vi "ConfigureNetworkAdapterByMAC.vi"(8 "error in (no error)":errorcluster, 10 "Network Adapter Settings":T1={"Adapter Mode"=1, "IsPrimary"=FALSE, "MACAddr"="", "IP Address Request Mode"=1, "IPAddr"="", "SubnetMask"="", "Gateway"="", "DNSServer"="", "Alias"=""} {"IP Address Request Mode" items=["Static"=1, "DHCP/Link Local"=2, "Link-Local Only"=4, "DHCP Only"=8]; "Adapter Mode" items=["Disabled"=1, "TCP/IP Ethernet"=2, "Deterministic"=4, "EtherCAT"=8, "TCP/IP WLAN Connect"=32, "TCP/IP WLAN Create"=64]}, 11 "Session in":refnum<k21>="localhost") -> (0 "error out":errorcluster, 2 "requires restart":bool, 3 "Session out":refnum<k21>)   [LabVIEW 2017, in "SystemInfoProcess.lvlib"]
uses:
  <vilib>/addons/SystemInfoProcess/SystemInfoProcess.lvlib
  <vilib>/addons/SystemInfoProcess/controls/NetworkAdapterSettings.ctl
  <vilib>/nisyscfg/Find Hardware.vi
  <vilib>/nisyscfg/Save Changes (Hardware).vi
  <vilib>/nisyscfg/Close (Hardware).vi
  <vilib>/nisyscfg/Close (Filter).vi
  <vilib>/nisyscfg/nisyscfg.lvlib
  <resource>/objmgr/niflexriosae.rc
  <resource>/objmgr/nicriosae.rc
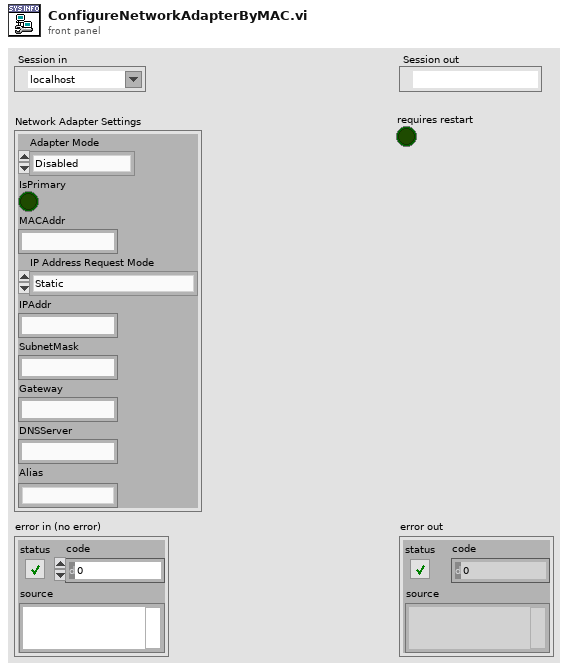
[diagram p1: front panel]
types:
  T1 = typedef "SystemInfoProcess.lvlib/NetworkAdapterSettings.ctl" = cluster{"Adapter Mode":u32, "IsPrimary":bool, "MACAddr":string, "IP Address Request Mode":u32, "IPAddr":string, "SubnetMask":string, "Gateway":string, "DNSServer":string, "Alias":string}
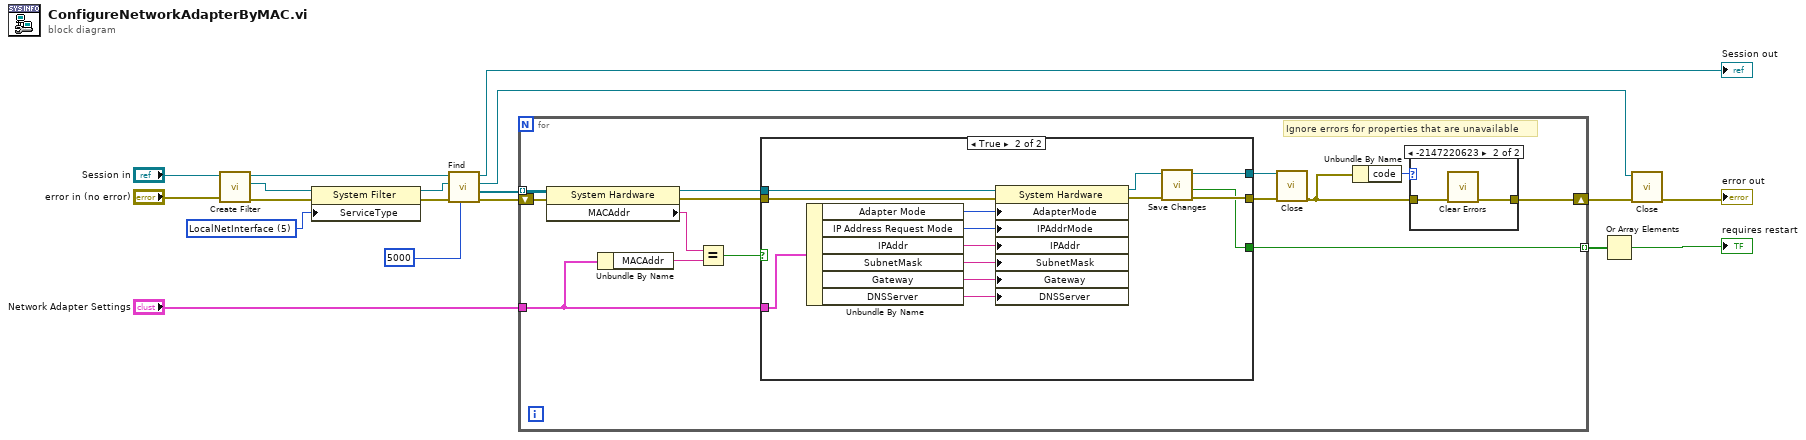
[diagram p0: block diagram]
diagram:
  w17 = u32 5 items=["mDnsNiTcp", "mDnsNiRealtime", "mDnsNiSysapi", "mDnsNiHttp", "LocalSystem", "LocalNetInterface", "LocalTimeKeeper", "LocalTimeSource", "mDnsLxi"] ("Service Type")
  n1 = call <vilib>:"Create Filter.vi"("error in (no error)"="error in (no error)", "Session in"="Session in") -> ("error out"=w16:errorcluster, "Filter out"=w18:refnum<k20>, "Session out"=w14:refnum<k21>)  [unwired: 7 in]
  n2 = property class="System Filter"(reference=w18, error in=w16, "ServiceType"=w17) -> (reference out=w13:refnum<k20>, error out=w15:errorcluster)
  n3 = call-poly <vilib>:"Find.vi"("Remote Timeout (300,000 ms)"=u32 5000 ("Timeout (milliseconds)"), "error in (no error)"=w15, "Filter in"=w13, "Session in"=w14) -> ("error out"=w11:errorcluster, "Resources out"=w12:refnum<k20>[], "Filter out"=w10:refnum<k20>, "Session out"=→"Session out":refnum<k21>)  [unwired: 4 in]
  n4 = for {
    tunnel: w12 -> [w31] mode=indexing
    shift-right: [w29] -> w8
    shift-left: w11 -> [w32]
    tunnel: "Network Adapter Settings" -> [w23]
    tunnel: [w19] -> w9 mode=indexing
    # "Ignore errors for properties that are unavailable"
    n5 = property class="System Hardware"(reference=w31, error in=w32) -> (reference out=w28:refnum<k20>, error out=w27:errorcluster, "MACAddr"=w26:string)
    n6 = Unbundle By Name(w23) -> ("MACAddr"=w25:string)
    n7 = Equal?(x=w26, y=w25) -> (x = y?=w24:bool)
    n8 = case shown="True" w24 {
      tunnel: w28 -> [w34 w48]
      tunnel: w27 -> [w33 w47]
      tunnel: [w34 w36] -> w21
      tunnel: [w33 w37] -> w22
      tunnel: w23 -> [_ w46]
      tunnel: [_ w35] -> w19
      frame False {
      }
      frame True {
        n9 = Unbundle By Name(w46) -> ("Adapter Mode"=w45:u32, "IP Address Request Mode"=w44:u32, "IPAddr"=w43:string, "SubnetMask"=w42:string, "Gateway"=w41:string, "DNSServer"=w40:string)
        n10 = property class="System Hardware"(reference=w48, error in=w47, "AdapterMode"=w45, "IPAddrMode"=w44, "IPAddr"=w43, "SubnetMask"=w42, "Gateway"=w41, "DNSServer"=w40) -> (reference out=w38:refnum<k20>, error out=w39:errorcluster)
        n11 = call-poly <vilib>:"Save Changes.vi"("error in (no error)"=w39, "Resource in"=w38) -> ("error out"=w37:errorcluster, "Changes Require Restart"=w35:bool, "Resource out"=w36:refnum<k20>)  [unwired: 6 in, 1 out]
      }
    }
    n12 = call-poly <vilib>:"Close.vi"("error in (no error)"=w22, "Resource in"=w21) -> ("error out"=w20:errorcluster)  [unwired: 9 in]
    n13 = Unbundle By Name(w20) -> ("code"=w30:i32)
    n14 = case shown="-2147220623" w30 {
      tunnel: [w49 w51] -> w29
      tunnel: w20 -> [w49 w50]
      frame 0, Default {
      }
      frame -2147220623 {
        n15 = call <vilib>:"Clear Errors.vi"("error in (no error)"=w50) -> ("error out"=w51:errorcluster)  [unwired: 5 in, 1 out]
      }
    }
  }
  n16 = Or Array Elements(Boolean array=w9) -> (logical OR=→"requires restart":bool)
  n17 = call-poly <vilib>:"Close.vi"("error in (no error)"=w8, "Filter in"=w10) -> ("error out"=→"error out":errorcluster)  [unwired: 9 in]
